vi "Test RoundTrip ComplexClusters.vi"(8 "error in (no error)":errorcluster) -> (0 "error out":errorcluster)   [LabVIEW 2013]
uses:
  <vilib>/addons/_JKI Toolkits/Caraya/classes/Test/Test.lvclass
  <vilib>/addons/_JKI Toolkits/Caraya/classes/Assert/Assert.lvclass
  src/JKI JSON Serialization.lvlib
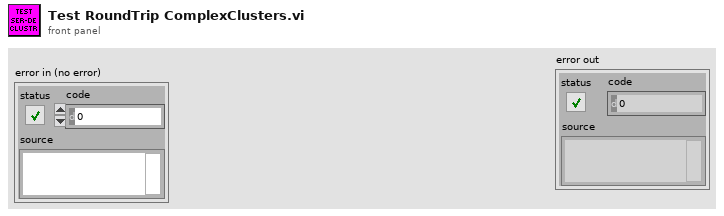
[diagram p1: front panel]
types:
  T1 = cluster{"Nested":cluster{"Nested.A":enum16{"test", "test1", "test2"}, "Nested.Bool":bool, "Array":dbl[]}, "A":enum16{"test", "test1", "test2"}, "Bool":bool}
  T2 = cluster{"Nested.A":enum16{"test", "test1", "test2"}, "Nested.Bool":bool, "Array":dbl[]}
  T3 = cluster{string, "Nested.Bool":bool, "Array":dbl[]}
  T4 = cluster{cluster{u16, "Nested.Bool":bool, "Array":dbl[]}, u16, "Bool":bool}
  T5 = cluster{cluster{string, "Nested.Bool":bool, "Array":dbl[]}, string, "Bool":bool}
  T6 = cluster{cluster{u16, "Nested.Bool":bool, "Array":dbl[]}, string, "Bool":bool}
  T7 = cluster{cluster{u16, "Nested.Bool":bool}, string, "Array":dbl[]}
  T8 = cluster{cluster{u16, "Nested.Bool":bool}, string}
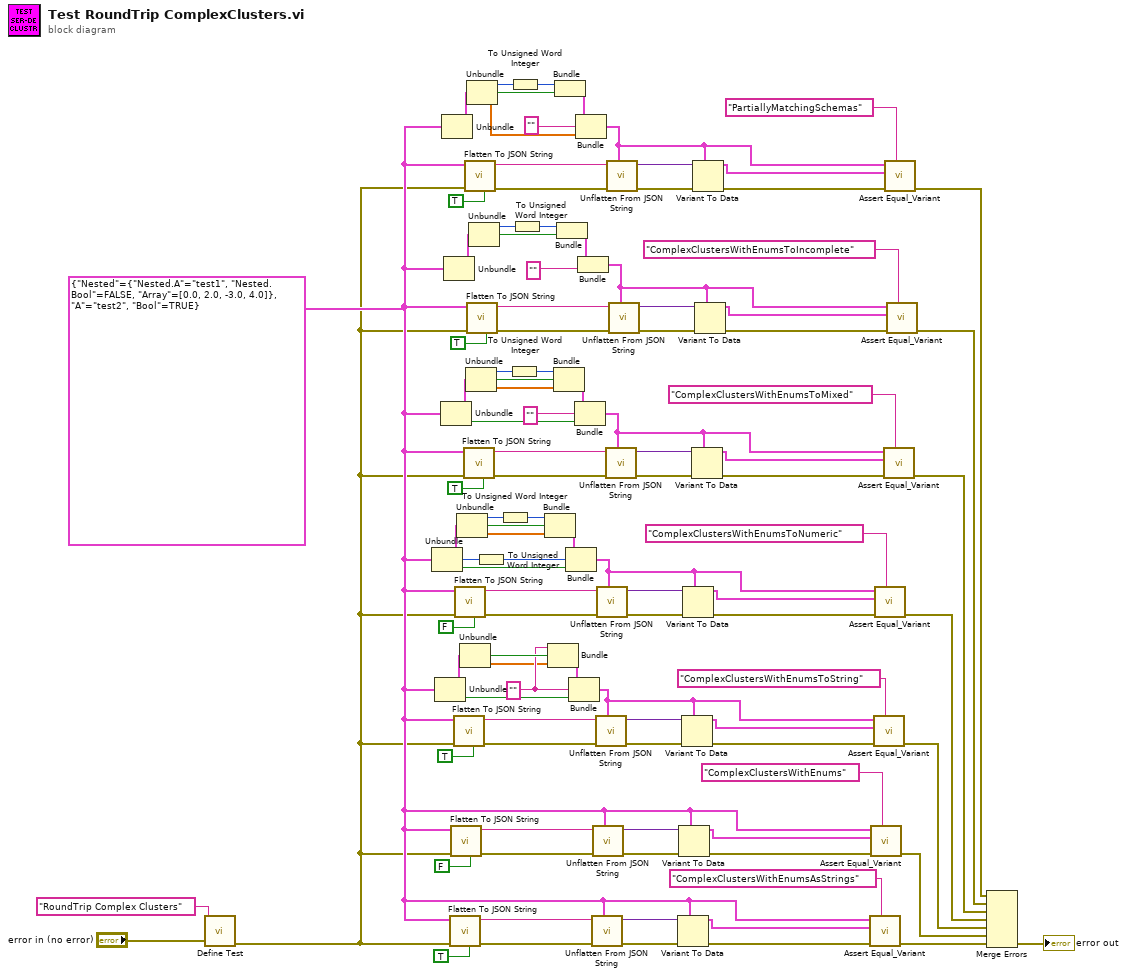
[diagram p0: block diagram]
diagram:
  w56 = ""
  w4 = T1 {"Nested"={"Nested.A"=enum."test1", "Nested.Bool"=FALSE, "Array"=[0.0, 2.0, -3.0, 4.0]}, "A"=enum."test2", "Bool"=TRUE}
  n1 = call <vilib>:"Define Test.vi"("error in (no error)"="error in (no error)", "Label (VI Title)"="RoundTrip Complex Clusters") -> ("error out"=w3:errorcluster)  [unwired: 9 in]
  n2 = Unbundle(w4) -> ("Nested"=w66:T2, "A"=w69:enum16{"test", "test1", "test2"}, "Bool"=w67:bool)
  n3 = Unbundle(w4) -> ("Nested"=w59:T2, "Bool"=w58:bool)  [unwired: 1 out]
  n4 = Unbundle(w4) -> ("Nested"=w51:T2, "Bool"=w50:bool)  [unwired: 1 out]
  n5 = Unbundle(w4) -> ("Nested"=w15:T2)  [unwired: 2 out]
  n6 = Unbundle(w4) -> ("Nested"=w25:T2)  [unwired: 2 out]
  n7 = call "Flatten To JSON String.vi"("Enums As String (F)"=TRUE, "error in (no error)"=w3, "Variant"=w4) -> ("error out"=w104:errorcluster, "JSON String"=w103:string)  [unwired: 7 in]
  n8 = call "Flatten To JSON String.vi"("Enums As String (F)"=FALSE, "error in (no error)"=w3, "Variant"=w4) -> ("error out"=w91:errorcluster, "JSON String"=w92:string)  [unwired: 7 in]
  n9 = call "Flatten To JSON String.vi"("Enums As String (F)"=TRUE, "error in (no error)"=w3, "Variant"=w4) -> ("error out"=w74:errorcluster, "JSON String"=w75:string)  [unwired: 7 in]
  n10 = call "Flatten To JSON String.vi"("Enums As String (F)"=FALSE, "error in (no error)"=w3, "Variant"=w4) -> ("error out"=w87:errorcluster, "JSON String"=w86:string)  [unwired: 7 in]
  n11 = Unbundle(w66) -> ("Nested.A"=w63:enum16{"test", "test1", "test2"}, "Nested.Bool"=w64:bool, "Array"=w37:dbl[])
  n12 = Unbundle(w59) -> ("Nested.Bool"=w61:bool, "Array"=w36:dbl[])  [unwired: 1 out]
  n13 = call "Flatten To JSON String.vi"("Enums As String (F)"=TRUE, "error in (no error)"=w3, "Variant"=w4) -> ("error out"=w42:errorcluster, "JSON String"=w43:string)  [unwired: 7 in]
  n14 = call "Flatten To JSON String.vi"("Enums As String (F)"=TRUE, "error in (no error)"=w3, "Variant"=w4) -> ("error out"=w7:errorcluster, "JSON String"=w8:string)  [unwired: 7 in]
  n15 = Unbundle(w51) -> ("Nested.A"=w54:enum16{"test", "test1", "test2"}, "Nested.Bool"=w53:bool, "Array"=w38:dbl[])
  n16 = Unbundle(w15) -> ("Nested.A"=w18:enum16{"test", "test1", "test2"}, "Nested.Bool"=w17:bool, "Array"=w2:dbl[])
  n17 = call "Flatten To JSON String.vi"("Enums As String (F)"=TRUE, "error in (no error)"=w3, "Variant"=w4) -> ("error out"=w33:errorcluster, "JSON String"=w32:string)  [unwired: 7 in]
  n18 = Unbundle(w25) -> ("Nested.A"=w22:enum16{"test", "test1", "test2"}, "Nested.Bool"=w23:bool)  [unwired: 1 out]
  n19 = To Unsigned Word Integer(number=w69) -> (unsigned 16bit integer=w68:u16)
  n20 = To Unsigned Word Integer(number=w63) -> (unsigned 16bit integer=w62:u16)
  n21 = To Unsigned Word Integer(number=w54) -> (unsigned 16bit integer=w55:u16)
  n22 = To Unsigned Word Integer(number=w18) -> (unsigned 16bit integer=w19:u16)
  n23 = To Unsigned Word Integer(number=w22) -> (unsigned 16bit integer=w21:u16)
  n24 = Bundle(w62, "Nested.Bool"=w64, "Array"=w37) -> (w65:cluster{u16, "Nested.Bool":bool, "Array":dbl[]})  [unwired: 1 in]
  n25 = Bundle(w56, "Nested.Bool"=w61, "Array"=w36) -> (w60:T3)  [unwired: 1 in]
  n26 = Bundle(w55, "Nested.Bool"=w53, "Array"=w38) -> (w52:cluster{u16, "Nested.Bool":bool, "Array":dbl[]})  [unwired: 1 in]
  n27 = Bundle(w19, "Nested.Bool"=w17) -> (w16:cluster{u16, "Nested.Bool":bool})  [unwired: 1 in]
  n28 = Bundle(w21, "Nested.Bool"=w23) -> (w24:cluster{u16, "Nested.Bool":bool})  [unwired: 1 in]
  n29 = Bundle(w65, w68, "Bool"=w67) -> (w70:T4)  [unwired: 1 in]
  n30 = Bundle(w60, w56, "Bool"=w58) -> (w57:T5)  [unwired: 1 in]
  n31 = Bundle(w52, "", "Bool"=w50) -> (w49:T6)  [unwired: 1 in]
  n32 = Bundle(w16, "", "Array"=w2) -> (w14:T7)  [unwired: 1 in]
  n33 = Bundle(w24, "") -> (w26:T8)  [unwired: 1 in]
  n34 = call "Unflatten From JSON String.vi"("Type and Defaults"=w4, "error in (no error)"=w104, "JSON String"=w103) -> ("error out"=w99:errorcluster, "Variant"=w101:variant)  [unwired: 7 in]
  n35 = call "Unflatten From JSON String.vi"("Type and Defaults"=w4, "error in (no error)"=w91, "JSON String"=w92) -> ("error out"=w96:errorcluster, "Variant"=w94:variant)  [unwired: 7 in]
  n36 = call "Unflatten From JSON String.vi"("Type and Defaults"=w57, "error in (no error)"=w74, "JSON String"=w75) -> ("error out"=w79:errorcluster, "Variant"=w77:variant)  [unwired: 7 in]
  n37 = call "Unflatten From JSON String.vi"("Type and Defaults"=w70, "error in (no error)"=w87, "JSON String"=w86) -> ("error out"=w82:errorcluster, "Variant"=w84:variant)  [unwired: 7 in]
  n38 = call "Unflatten From JSON String.vi"("Type and Defaults"=w49, "error in (no error)"=w42, "JSON String"=w43) -> ("error out"=w47:errorcluster, "Variant"=w45:variant)  [unwired: 7 in]
  n39 = call "Unflatten From JSON String.vi"("Type and Defaults"=w14, "error in (no error)"=w7, "JSON String"=w8) -> ("error out"=w12:errorcluster, "Variant"=w10:variant)  [unwired: 7 in]
  n40 = call "Unflatten From JSON String.vi"("Type and Defaults"=w26, "error in (no error)"=w33, "JSON String"=w32) -> ("error out"=w28:errorcluster, "Variant"=w30:variant)  [unwired: 7 in]
  n41 = Variant To Data(error in=w99, type=w4, Variant=w101) -> (data=w100:T1, error out=w98:errorcluster)
  n42 = Variant To Data(error in=w96, type=w4, Variant=w94) -> (data=w95:T1, error out=w97:errorcluster)
  n43 = Variant To Data(error in=w79, type=w57, Variant=w77) -> (data=w78:T5, error out=w80:errorcluster)
  n44 = Variant To Data(error in=w82, type=w70, Variant=w84) -> (data=w83:T4, error out=w81:errorcluster)
  n45 = Variant To Data(error in=w47, type=w49, Variant=w45) -> (data=w46:T6, error out=w48:errorcluster)
  n46 = Variant To Data(error in=w12, type=w14, Variant=w10) -> (data=w11:T7, error out=w13:errorcluster)
  n47 = Variant To Data(error in=w28, type=w26, Variant=w30) -> (data=w29:T8, error out=w27:errorcluster)
  n48 = call <vilib>:"Assert Equal_Variant.vi"("Label"="ComplexClustersWithEnumsAsStrings", "error in (no error)"=w98, "Y"=w100, "X"=w4) -> ("error out"=w106:errorcluster)  [unwired: 7 in]
  n49 = call <vilib>:"Assert Equal_Variant.vi"("Label"="ComplexClustersWithEnums", "error in (no error)"=w97, "Y"=w95, "X"=w4) -> ("error out"=w89:errorcluster)  [unwired: 7 in]
  n50 = call <vilib>:"Assert Equal_Variant.vi"("Label"="ComplexClustersWithEnumsToString", "error in (no error)"=w80, "Y"=w78, "X"=w57) -> ("error out"=w72:errorcluster)  [unwired: 7 in]
  n51 = call <vilib>:"Assert Equal_Variant.vi"("Label"="ComplexClustersWithEnumsToNumeric", "error in (no error)"=w81, "Y"=w83, "X"=w70) -> ("error out"=w71:errorcluster)  [unwired: 7 in]
  n52 = call <vilib>:"Assert Equal_Variant.vi"("Label"="ComplexClustersWithEnumsToMixed", "error in (no error)"=w48, "Y"=w46, "X"=w49) -> ("error out"=w40:errorcluster)  [unwired: 7 in]
  n53 = call <vilib>:"Assert Equal_Variant.vi"("Label"="PartiallyMatchingSchemas", "error in (no error)"=w13, "Y"=w11, "X"=w14) -> ("error out"=w1:errorcluster)  [unwired: 7 in]
  n54 = call <vilib>:"Assert Equal_Variant.vi"("Label"="ComplexClustersWithEnumsToIncomplete", "error in (no error)"=w27, "Y"=w29, "X"=w26) -> ("error out"=w20:errorcluster)  [unwired: 7 in]
  n55 = Merge Errors(w1, w20, w40, w71, w72, w89, w106) -> (→"error out":errorcluster)
